vi "Check for Duplicate Destinations.vi"(8 "error in (no error)":errorcluster, 11 "Destinations":string[](array[string])) -> (0 "error out":errorcluster, 3 "Duplicate Indices":i32[](array[numeric]))   [LabVIEW 2016, in "System Mapping Tool.lvlib"]
uses:
  System Mapping Tool.lvlib
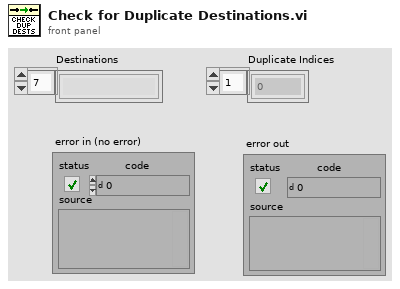
[diagram p1: front panel]
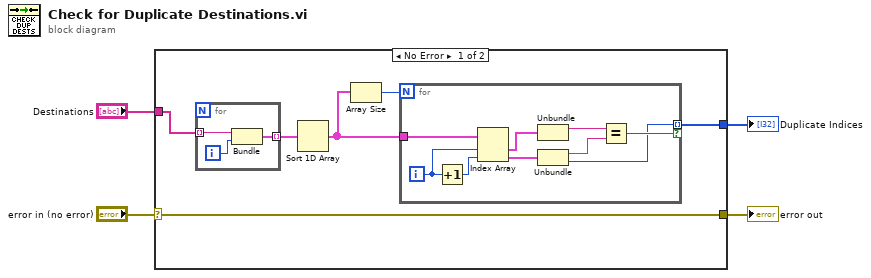
[diagram p0: block diagram]
diagram:
  n1 = case shown="No Error" "error in (no error)" {
    selector: "error in (no error)" -> [w8 w23]
    tunnel: [w8 w23] -> w3
    tunnel: "Destinations" -> [w10 _]
    tunnel: [w5 _] -> w1
    frame No Error {
      n2 = for {
        tunnel: w10 -> [w21] mode=indexing
        tunnel: [w20] -> w9 mode=indexing
        i -> [w22]
        n3 = Bundle("String"=w21, w22) -> (w20:cluster{"String":string, i32})  [unwired: 1 in]
      }
      n4 = Sort 1D Array(array=w9) -> (sorted array=w7:cluster{"String":string, i32}[])
      n5 = Array Size(array=w7) -> (size(s)=w6:i32)
      n6 = for {
        N: w6 -> [_]
        tunnel: w7 -> [w19]
        tunnel: [w12] -> w5 mode=indexing if=w14
        i -> [w11]
        n7 = Increment(x=w11) -> (x+1=w13:i32)
        n8 = Index Array(array=w19, index #1=w11, index #2=w13) -> (element #1=w17:cluster{"String":string, i32}, element #2=w18:cluster{"String":string, i32})
        n9 = Unbundle(w17) -> ("String"=w16:string)  [unwired: 1 out]
        n10 = Unbundle(w18) -> ("String"=w15:string, w12:i32)
        n11 = Equal?(x=w16, y=w15) -> (x = y?=w14:bool)
      }
    }
    frame Error {
    }
  }
  "Duplicate Indices" <- w1
  "error out" <- w3
